vi "Write Read Only.vi"(8 "error in (no error)":errorcluster, 10 "Read Only":bool, 11 "Abs_Value in":refnum<class "Abs_Value.lvclass">) -> (0 "error out":errorcluster, 3 "Abs_Value out":refnum<class "Abs_Value.lvclass">)   [LabVIEW 2021, in "Abs_Value.lvclass"]
uses:
  Abs_Value.lvclass
  Abs_Value.lvclass/Abs_Value.ctl
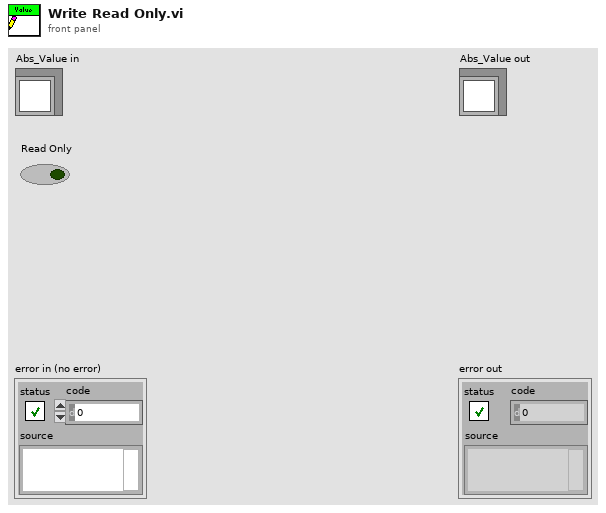
[diagram p1: front panel]
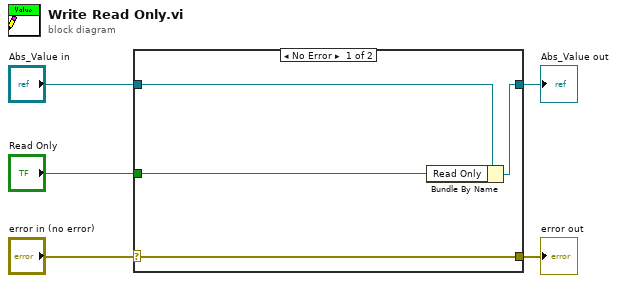
[diagram p0: block diagram]
diagram:
  n1 = case shown="No Error" "error in (no error)" {
    selector: "error in (no error)" -> [w9 w10]
    tunnel: [w9 w10] -> w4
    tunnel: [w7 w11] -> w2
    tunnel: "Abs_Value in" -> [w8 w11]
    tunnel: "Read Only" -> [w6 _]
    frame No Error {
      n2 = Bundle By Name(cluster=w8, "Read Only"=w6) -> (w7:refnum<class "Abs_Value.lvclass">)
    }
    frame Error {
    }
  }
  "error out" <- w4
  "Abs_Value out" <- w2
